vi "Calculate Driving Direction1.vi"(4 "angle":dbl, 5 "Tank2":dbl[](array[numeric]), 6 "Identity":bool, 7 "Tank1":dbl[](array[numeric]), 8 "error in (no error)":errorcluster, 10 "obstacle angles (rad)":dbl[](array[numeric]), 11 "obstacle distances (m)":dbl[](array[numeric])) -> (0 "error out":errorcluster, 3 "steering frame velocity":dbl[](array[numeric]))   [LabVIEW 2012]
doc: "Calculates the velocity vector of the robot required to avoid obstacles, based on the scanned data."
uses:
  <vilib>/robotics/Obstacle Avoidance/Simple Vector Field Histogram/Panic Range.ctl
  <vilib>/Utility/AngleManip/Degrees to Radians (Scalar DBL).vi
  <vilib>/robotics/Obstacle Avoidance/Simple Vector Field Histogram/NI_Robotics_Simple Vector Field Histogram.lvlib
  <vilib>/Utility/AngleManip/NI_AngleManipulation.lvlib
panel:
  out ".not. x?":bool
  in  "dir1":dbl
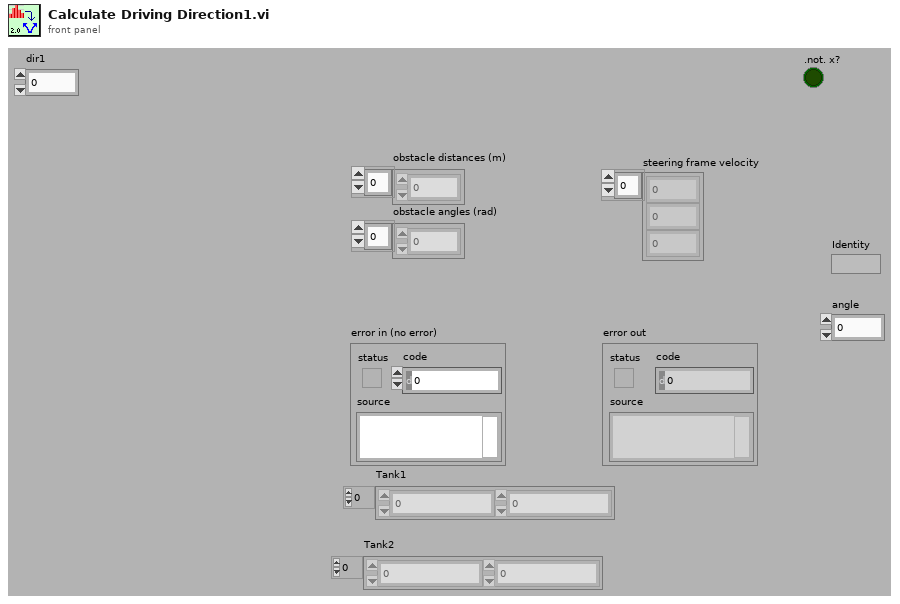
[diagram p1: front panel]
types:
  T1 = typedef "NI_Robotics_Simple Vector Field Histogram.lvlib/Panic Range.ctl" = cluster{"panic threshold distance (0)":dbl, "panic threshold angle (0)":dbl}
  T2 = typedef "NI_Robotics_Simple Vector Field Histogram.lvlib/Obstacle Description.ctl" = cluster{"angle to obstacle":dbl, "distance to obstacle":dbl}
  T3 = typedef "NI_Robotics_Simple Vector Field Histogram.lvlib/Gap Description.ctl" = cluster{"angle to gap":dbl, "size of gap":dbl}
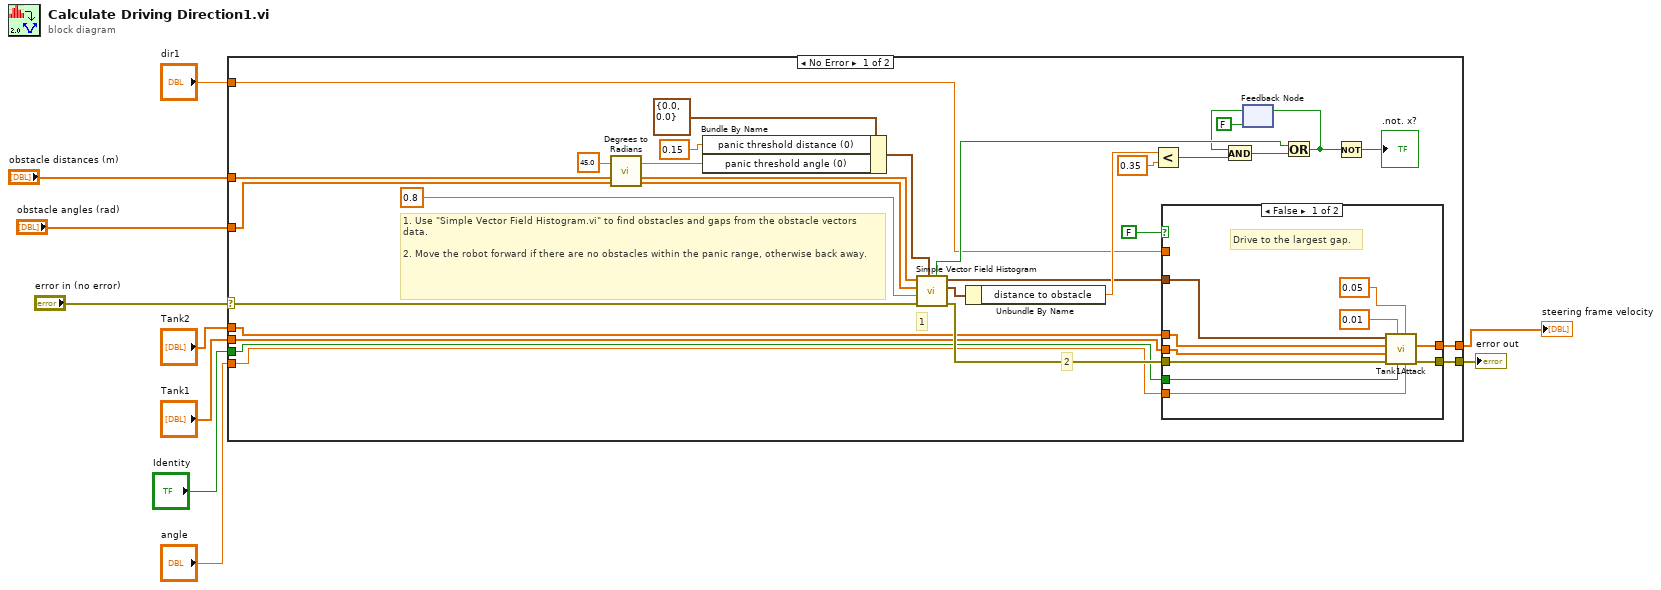
[diagram p0: block diagram]
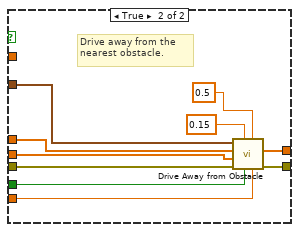
[diagram p2: hidden frame]
diagram:
  n1 = case shown="No Error" "error in (no error)" {
    selector: "error in (no error)" -> [w22 w60]
    tunnel: [w23 w60] -> w10
    tunnel: "obstacle distances (m)" -> [w21 _]
    tunnel: "obstacle angles (rad)" -> [w20 _]
    tunnel: [w19 _] -> w6
    tunnel: "Identity" -> [w17 _]
    tunnel: "angle" -> [w16 _]
    tunnel: "Tank1" -> [w15 _]
    tunnel: "Tank2" -> [w14 _]
    tunnel: "dir1" -> [w13 _]
    frame No Error {
      # "2"
      # "1"
      # "1. Use \"Simple Vector Field Histogram.vi\" to find obstacles and gaps from the obstacle vectors data.\n\n2. Move the robot forward if there are no obstacles within the panic range, otherwise back away."
      n2 = call-poly <vilib>:"Degrees to Radians.vi"("angle (deg)"=45.0 ("panic threshold angle (rad)")) -> ("angle (rad)"=w39:dbl)  [unwired: 2 in]
      n3 = Bundle By Name(cluster=T1 {"panic threshold distance (0)"=0.0, "panic threshold angle (0)"=0.0} ("panic range"), "panic threshold distance (0)"=0.15 ("panic threshold distance (m)"), "panic threshold angle (0)"=w39) -> (w27:T1)
      n4 = call <vilib>:"Simple Vector Field Histogram.vi"("panic range"=w27, "error in (no error)"=w22, "distance threshold"=0.8 ("distance threshold (m)"), "direction angles"=w20, "distances"=w21) -> ("error out"=w24:errorcluster, "nearest obstacle"=w29:T2, "largest gap"=w18:T3, "obstacle within panic range"=w34:bool)  [unwired: 2 in, 1 out]
      n5 = Unbundle By Name(w29) -> ("distance to obstacle"=w30:dbl)
      n6 = Less?(x=w30, y=0.35) -> (x < y?=w32:bool)
      n7 = case shown="False" FALSE {
        tunnel: w18 -> [w42 w57]
        tunnel: w24 -> [w48 w59]
        tunnel: [w49 w58] -> w23
        tunnel: [w44 w56] -> w19
        tunnel: w17 -> [w47 w53]
        tunnel: w16 -> [w43 w52]
        tunnel: w14 -> [w41 w51]
        tunnel: w15 -> [w40 w50]
        tunnel: w13 -> [_ _]
        frame False {
          # "Drive to the largest gap."
          n8 = call "Tank1Attack.vi"("angle"=w43, "max forward velocity (m/s)"=0.05, "find"=w47, "max angular velocity (rad/s)"=0.01, "error in (no error)"=w48, "Tank2"=w40, "Tank1"=w41, "gap"=w42) -> ("error out"=w49:errorcluster, "steering frame velocity"=w44:dbl[])  [unwired: 2 in]
        }
        frame True {
          # "Drive away from the nearest obstacle."
          n9 = call "Drive Away from Obstacle.vi"("angle"=w52, "max reverse velocity (m/s)"=0.5, "Find"=w53, "max angular velocity (rad/s)"=0.15, "error in (no error)"=w59, "Tank1"=w50, "Tank2"=w51, "gap"=w57) -> ("error out"=w58:errorcluster, "steering frame velocity"=w56:dbl[])  [unwired: 2 in]
        }
      }
      n10 = feedback #1(FALSE ("obstacle within panic range")) -> (w33:bool)
      n11 = And(x=w33, y=w32) -> (x .and. y?=w35:bool)
      n12 = Or(x=w34, y=w35) -> (x .or. y?=w37:bool)
      n13 = feedback-in #1(w37) -> ()
      n14 = Not(x=w37) -> (.not. x?=→".not. x?":bool)
    }
    frame Error {
    }
  }
  "error out" <- w10
  "steering frame velocity" <- w6
